vi "Display Console.vi"(8 "error in (no error)":errorcluster, 10 "Queues":T1, 11 "UE Data Container":T2) -> (0 "error out":errorcluster)   [LabVIEW 2017]
doc: "Uses for display current ATM status (Transaction/Message/CardReader).\n[Covers: UI3]"
uses:
  Shared Data/User Events/UE Data Container.ctl
  Error Handler/Controls/Error Data.ctl
  User Console/Controls/User Console - Transaction Enum.ctl
  Shared Data/Queues/Controls/Queues.ctl
  Controller/Controls/Controller CMD.ctl
  Configuration/Controls/Config CMD.ctl
  Controls/Display Data.ctl
panel:
  out "Card Read":bool
  out "Message Screen":string
  out "Current Transaction":string
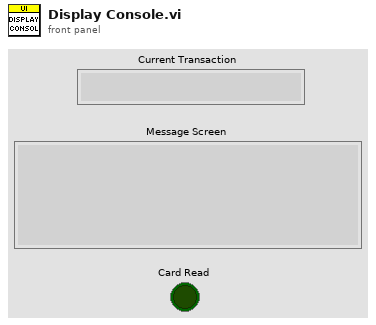
[diagram p1: front panel]
types:
  T1 = typedef "Queues.ctl" = cluster{"Controller":refnum<queue>, "Config":refnum<queue>, "Display Console":refnum<queue>}
  T2 = typedef "UE Data Container.ctl" = cluster{"Stop UE":refnum<user-event>, "Error UE":refnum<user-event>, "Deposit Change":refnum<user-event>, "Funds Change":refnum<user-event>, "Card Reader Change":refnum<user-event>, "Transaction Change":refnum<user-event>, "Keypad Screen Change":refnum<user-event>}
  T3 = typedef "Controller CMD.ctl" = cluster{"Command":enum16{"Idle", "Init", "Config Update", "Terminate", "Send Message", "Login Start", "Login Finish", "Balance", "Deposit", "Withdrawal", "Fast Cash Start", "Fast Cash Stop", "Keypad Proc", "Search Account"}, "Data":variant}
  T4 = enum16{"Idle", "Init", "Config Update", "Terminate", "Send Message", "Login Start", "Login Finish", "Balance", "Deposit", "Withdrawal", "Fast Cash Start", "Fast Cash Stop", "Keypad Proc", "Search Account"}
  T5 = typedef "Display Data.ctl" = cluster{"Transaction":string, "Message":string, "Card Read":bool}
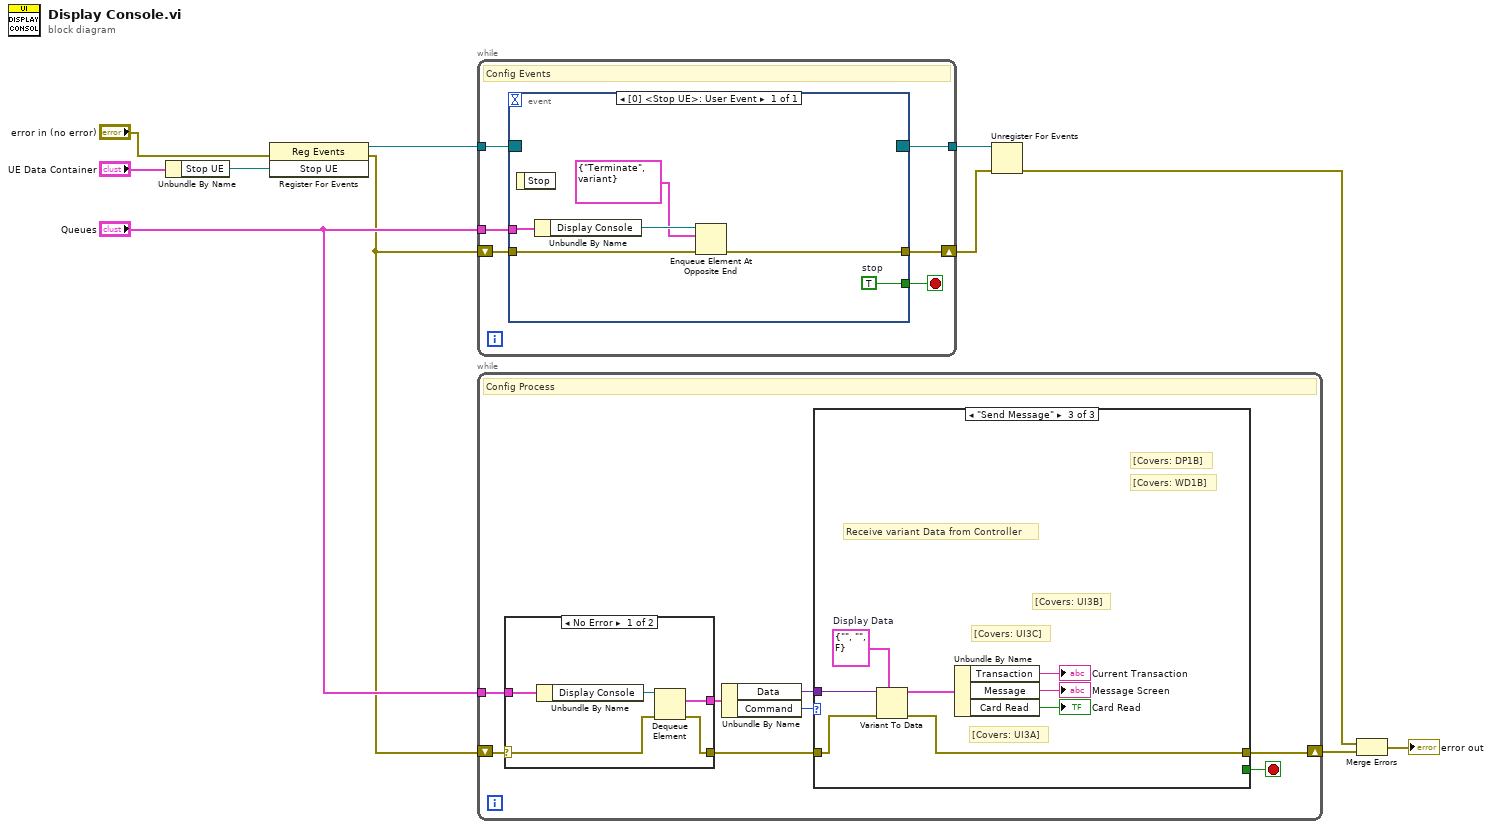
[diagram p0: block diagram]
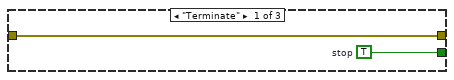
[diagram p2: hidden frame]
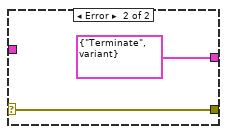
[diagram p4: hidden frame]
diagram:
  n1 = Unbundle By Name("UE Data Container") -> ("Stop UE"=w10:refnum<user-event>)
  n2 = register-events(error in="error in (no error)", w10) -> (reference out=w8:refnum<event-registration>, error out=w4:errorcluster)  [unwired: 1 in]
  n3 = while {
    tunnel: w8 -> [w17]
    tunnel: [w16] -> w7
    tunnel: "Queues" -> [w14]
    shift-right: [w12] -> w6
    shift-left: w4 -> [w13]
    stop <- w15 stop-if-true
    # "Config Events"
    n4 = event shown="[0] <Stop UE>: User Event" {
      selector: w17 -> [_]
      dyn-events: [_] -> w16
      timeout: _ -> [_]
      tunnel: [w23] -> w15
      tunnel: w14 -> [w22]
      tunnel: w13 -> [w20]
      tunnel: [w19] -> w12
      event User Event {
        w23 = TRUE  # stop
        n5 = event-data() -> ()  [unwired: 1 in, 1 out]
        n6 = Unbundle By Name(w22) -> ("Display Console"=w21:refnum<queue>)
        n7 = Enqueue Element At Opposite End(queue=w21, element=T3 {"Command"=enum."Terminate", "Data"=variant} ("Controller CMD"), error in (no error)=w20) -> (error out=w19:errorcluster)  [unwired: 1 in, 2 out]
      }
    }
  }
  n8 = while {
    tunnel: "Queues" -> [w31]
    shift-right: [w25] -> w3
    shift-left: w4 -> [w30]
    stop <- w24 stop-if-true
    # "Config Process"
    n9 = case shown="No Error" w30 {
      selector: w30 -> [w45 w49]
      tunnel: w31 -> [w47 _]
      tunnel: [w44 T3 {"Command"=enum."Terminate", "Data"=variant} ("Controller CMD")] -> w29
      tunnel: [w43 w49] -> w26
      frame No Error {
        n10 = Unbundle By Name(w47) -> ("Display Console"=w46:refnum<queue>)
        n11 = Dequeue Element(queue=w46, error in (no error)=w45) -> (element=w44:T3, error out=w43:errorcluster)  [unwired: 1 in, 2 out]
      }
      frame Error {
      }
    }
    n12 = Unbundle By Name(w29) -> ("Data"=w27:variant, "Command"=w28:T4)
    n13 = case shown="\"Send Message\"" w28 {
      tunnel: w27 -> [_ _ w42]
      tunnel: w26 -> [w33 w34 w36]
      tunnel: [w33 w34 w35] -> w25
      tunnel: [w32 _ _] -> w24
      frame "Terminate" {
        w32 = TRUE  # stop
      }
      frame "Idle", Default {
      }
      frame "Send Message" {
        w41 = T5 {"Transaction"="", "Message"="", "Card Read"=FALSE}  # Display Data
        # "[Covers: DP1B]"
        # "[Covers: WD1B]"
        # "Receive variant Data from Controller"
        # "[Covers: UI3C]"
        # "[Covers: UI3B]"
        # "[Covers: UI3A]"
        n14 = Variant To Data(error in=w36, type=w41, Variant=w42) -> (data=w40:T5, error out=w35:errorcluster)
        n15 = Unbundle By Name(w40) -> ("Transaction"=→"Current Transaction":string, "Message"=→"Message Screen":string, "Card Read"=→"Card Read":bool)
      }
    }
  }
  n16 = Unregister For Events(event registration refnum=w7, error in=w6) -> (error out=w2:errorcluster)
  n17 = Merge Errors(w2, w3) -> (→"error out":errorcluster)
